vi "hw3-4 topVI.vi"() -> ()   [LabVIEW 2014]
panel:
  out "change":bool
  in  "stop/start":bool
  out "negative":bool
  in  "ss":i32
  in  "mm":i32
  in  "hh":i32
  # ":"
  # ":"
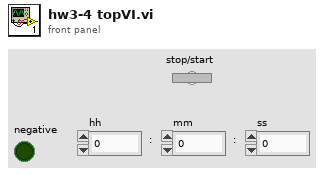
[diagram p1: front panel]
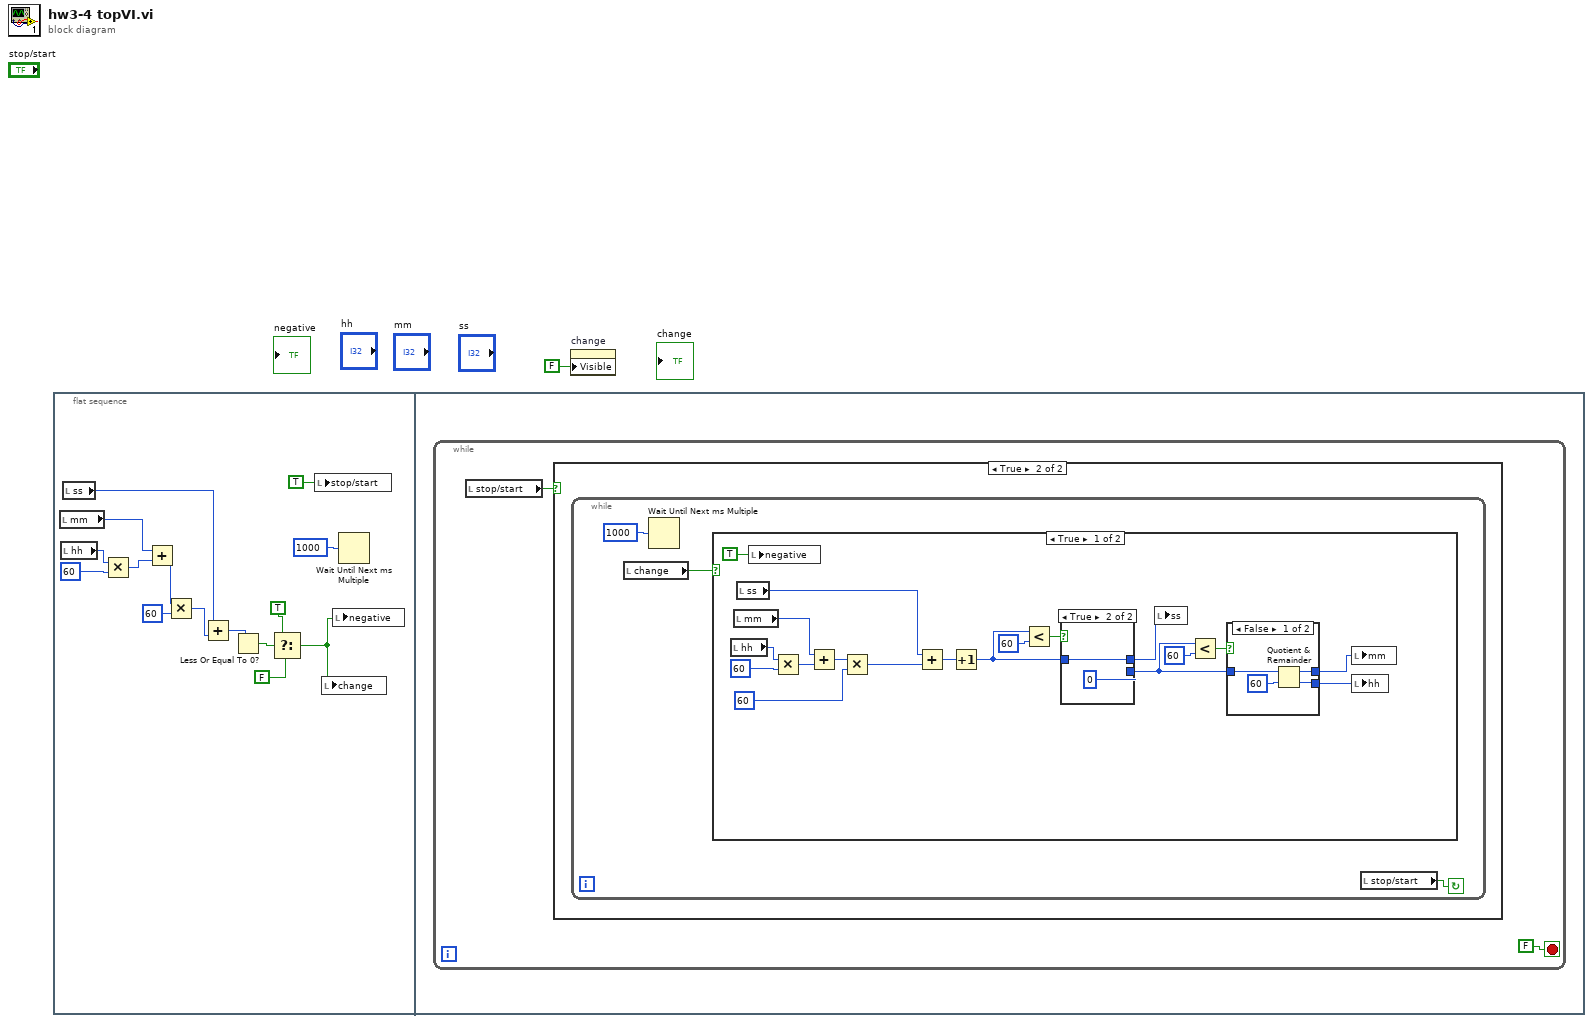
[diagram p0: block diagram]
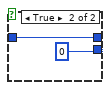
[diagram p3: hidden frame]
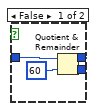
[diagram p4: hidden frame]
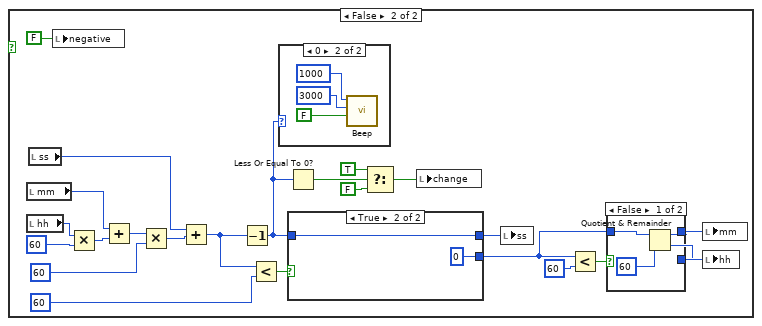
[diagram p5: hidden frame]
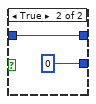
[diagram p7: hidden frame]
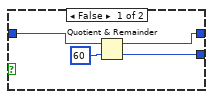
[diagram p8: hidden frame]
diagram:
  n1 = flat-sequence {
    frame #0 {
      n2 = local read "mm"() -> (w13:i32)
      n3 = local read "hh"() -> (w16:i32)
      n4 = local read "ss"() -> (w10:i32)
      n5 = Multiply(x=w16, y=60) -> (x*y=w14:i32)
      n6 = Add(x=w13, y=w14) -> (x+y=w12:i32)
      n7 = Multiply(x=w12, y=60) -> (x*y=w9:i32)
      n8 = Add(x=w10, y=w9) -> (x+y=w3:i32)
      n9 = Less Or Equal To 0?(x=w3) -> (x <= 0?=w2:bool)
      n10 = Select(t=TRUE, s=w2, f=FALSE) -> (s? t:f=w4:bool)
      n11 = local write "stop/start"(TRUE) -> ()
      n12 = local write "change"(w4) -> ()
      n13 = local write "negative"(w4) -> ()
      n14 = Wait Until Next ms Multiple(millisecond multiple=u32 1000) -> ()  [unwired: 1 out]
    }
    frame #1 {
      n15 = while {
        stop <- FALSE stop-if-true
        n16 = local read "stop/start"() -> (w17:bool)
        n17 = case shown="True" w17 {
          frame False {
          }
          frame True {
            n18 = while {
              stop <- w19 continue-if-true
              n19 = local read "change"() -> (w21:bool)
              n20 = Wait Until Next ms Multiple(millisecond multiple=u32 1000) -> ()  [unwired: 1 out]
              n21 = case shown="True" w21 {
                frame True {
                  n22 = local read "hh"() -> (w40:i32)
                  n23 = local read "mm"() -> (w37:i32)
                  n24 = local read "ss"() -> (w34:i32)
                  n25 = local write "negative"(TRUE) -> ()
                  n26 = Multiply(x=w40, y=60) -> (x*y=w38:i32)
                  n27 = Add(x=w37, y=w38) -> (x+y=w36:i32)
                  n28 = Multiply(x=w36, y=60) -> (x*y=w33:i32)
                  n29 = Add(x=w34, y=w33) -> (x+y=w24:i32)
                  n30 = Increment(x=w24) -> (x+1=w23:i32)
                  n31 = Less?(x=w23, y=60) -> (x < y?=w30:bool)
                  n32 = case shown="True" w30 {
                    tunnel: w23 -> [w50 w52]
                    tunnel: [w48 w52] -> w26
                    tunnel: [w47 0] -> w32
                    frame False {
                      n33 = Quotient & Remainder(x=w50, y=60) -> (x-y*floor(x/y)=w48:i32, floor(x/y)=w47:i32)
                    }
                    frame True {
                    }
                  }
                  n34 = local write "ss"(w26) -> ()
                  n35 = Less?(x=w32, y=60) -> (x < y?=w29:bool)
                  n36 = case shown="False" w29 {
                    tunnel: w32 -> [w44 w46]
                    tunnel: [w41 0] -> w27
                    tunnel: [w42 w46] -> w25
                    frame False {
                      n37 = Quotient & Remainder(x=w44, y=60) -> (x-y*floor(x/y)=w42:i32, floor(x/y)=w41:i32)
                    }
                    frame True {
                    }
                  }
                  n38 = local write "mm"(w25) -> ()
                  n39 = local write "hh"(w27) -> ()
                }
                frame False {
                  n40 = local read "mm"() -> (w72:i32)
                  n41 = local read "hh"() -> (w75:i32)
                  n42 = local read "ss"() -> (w69:i32)
                  n43 = local write "negative"(FALSE) -> ()
                  n44 = Multiply(x=w75, y=60) -> (x*y=w73:i32)
                  n45 = Add(x=w72, y=w73) -> (x+y=w71:i32)
                  n46 = Multiply(x=w71, y=60) -> (x*y=w68:i32)
                  n47 = Add(x=w69, y=w68) -> (x+y=w56:i32)
                  n48 = Decrement(x=w56) -> (x-1=w54:i32)
                  n49 = Less?(x=w56, y=60) -> (x < y?=w65:bool)
                  n50 = case shown="0" w54 {
                    frame Default {
                    }
                    frame 0 {
                      n51 = call <vilib>:"Beep.vi"("use system alert? (T)"=FALSE, "duration (msec)"=u32 3000, "frequency (Hz)"=u32 1000) -> ()  [unwired: 9 in]
                    }
                  }
                  n52 = Less Or Equal To 0?(x=w54) -> (x <= 0?=w55:bool)
                  n53 = case shown="True" w65 {
                    tunnel: w54 -> [w88 w90]
                    tunnel: [w86 w90] -> w61
                    tunnel: [w85 0] -> w67
                    frame False {
                      n54 = Quotient & Remainder(x=w88, y=60) -> (x-y*floor(x/y)=w86:i32, floor(x/y)=w85:i32)
                    }
                    frame True {
                    }
                  }
                  n55 = Select(t=TRUE, s=w55, f=FALSE) -> (s? t:f=w57:bool)
                  n56 = local write "change"(w57) -> ()
                  n57 = local write "ss"(w61) -> ()
                  n58 = Less?(x=w67, y=60) -> (x < y?=w64:bool)
                  n59 = case shown="False" w64 {
                    tunnel: w67 -> [w82 w84]
                    tunnel: [w79 0] -> w62
                    tunnel: [w80 w84] -> w60
                    frame False {
                      n60 = Quotient & Remainder(x=w82, y=60) -> (x-y*floor(x/y)=w80:i32, floor(x/y)=w79:i32)
                    }
                    frame True {
                    }
                  }
                  n61 = local write "mm"(w60) -> ()
                  n62 = local write "hh"(w62) -> ()
                }
              }
              n63 = local read "stop/start"() -> (w19:bool)
            }
          }
        }
      }
    }
  }
  n64 = property on="change" class="Bool (strict)"("Visible"=FALSE) -> ()  [unwired: 2 in, 2 out]
